vi "Get Valid Properties.vi"(0 "SigMan in":refnum<class "SignalManager.lvclass">, 11 "error in (no error)":errorcluster) -> (4 "SigMan out":refnum<class "SignalManager.lvclass">, 8 "Properties":string[](array[string]), 15 "error out":errorcluster)   [LabVIEW 2020, in "SignalManager.lvclass"]
uses:
  SignalManager.lvclass
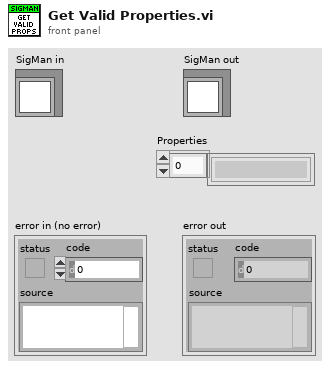
[diagram p1: front panel]
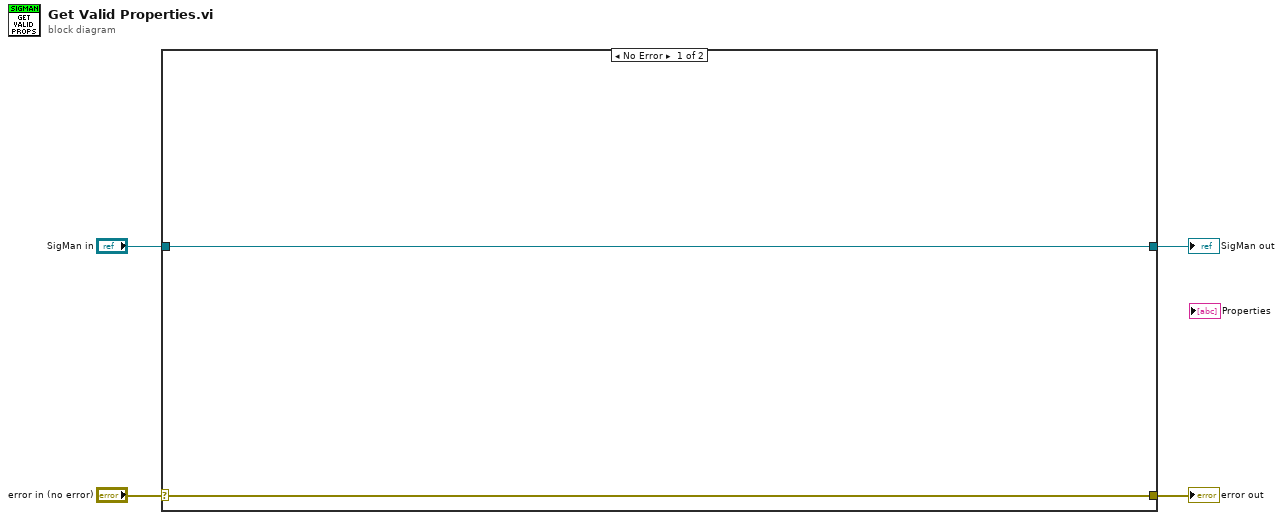
[diagram p0: block diagram]
diagram:
  n1 = case shown="No Error" "error in (no error)" {
    selector: "error in (no error)" -> [w6 w8]
    tunnel: [w6 w8] -> w3
    tunnel: [w5 w7] -> w1
    tunnel: "SigMan in" -> [w5 w7]
    frame No Error {
    }
    frame Error {
    }
  }
  "error out" <- w3
  "SigMan out" <- w1
